vi "getPointFromLineIntersection.vi"(6 "b2":dbl, 7 "b1":dbl, 8 "error in (no error)":errorcluster, 9 "a2":dbl, 10 "a1":dbl, 11 "Utilities in":refnum<class "Utilities.lvclass">) -> (0 "error out":errorcluster, 1 "y_intersection":dbl, 2 "x_intersection":dbl, 3 "Utilities out":refnum<class "Utilities.lvclass">)   [LabVIEW 2023, in "Utilities.lvclass"]
uses:
  Utilities.lvclass
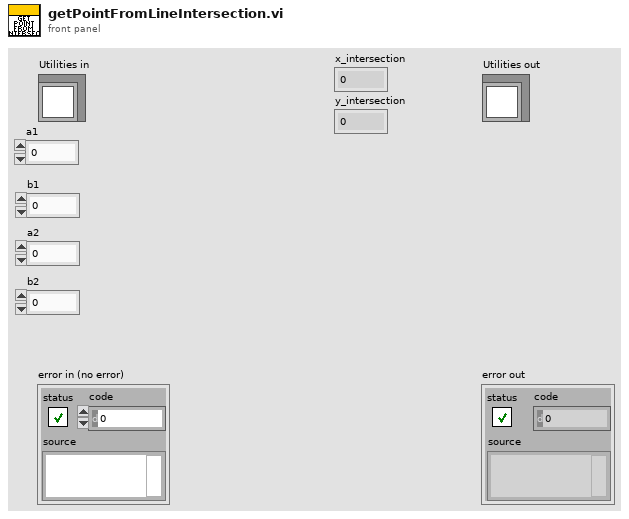
[diagram p1: front panel]
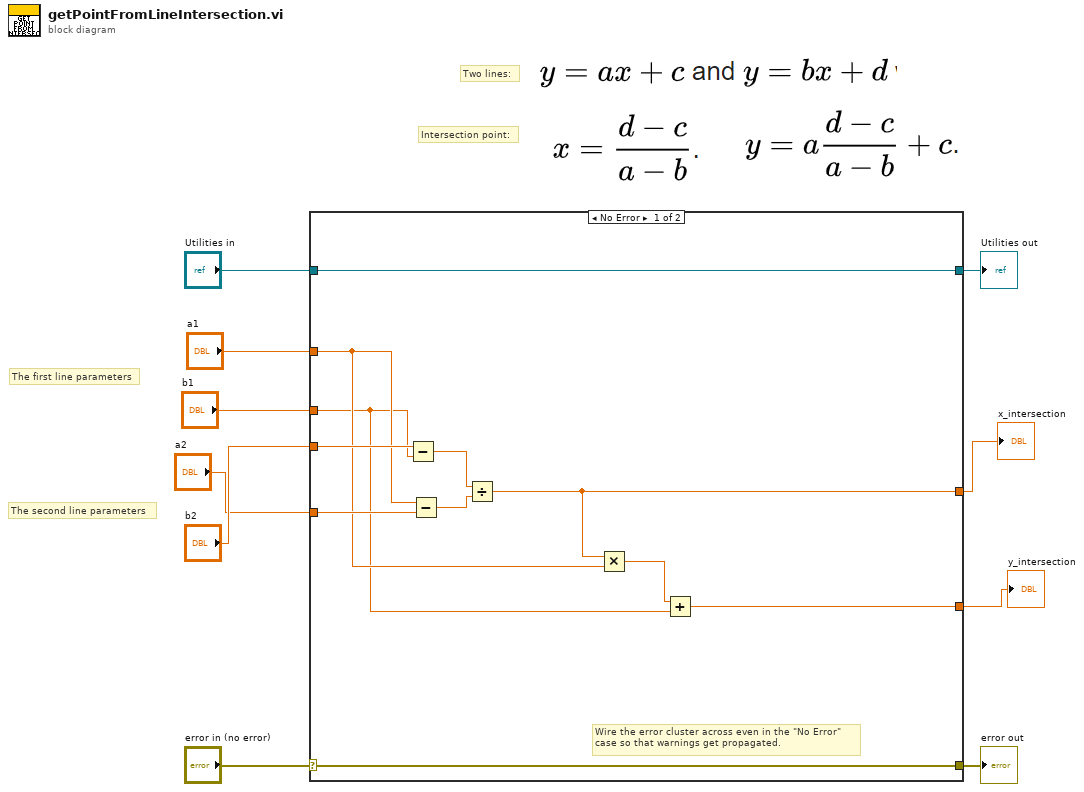
[diagram p0: block diagram]
diagram:
  # "The second line parameters"
  # "The first line parameters"
  # "Intersection point:"
  # "Two lines:"
  n1 = case shown="No Error" "error in (no error)" {
    selector: "error in (no error)" -> [w20 w23]
    tunnel: [w20 w23] -> w9
    tunnel: [w21 w22] -> w7
    tunnel: "Utilities in" -> [w21 w22]
    tunnel: "b2" -> [w19 _]
    tunnel: "b1" -> [w12 _]
    tunnel: "a1" -> [w14 _]
    tunnel: "a2" -> [w18 _]
    tunnel: [w15 _] -> w2
    tunnel: [w11 _] -> w1
    frame No Error {
      # "Wire the error cluster across even in the \"No Error\"\ncase so that warnings get propagated."
      n2 = Subtract(x=w19, y=w12) -> (x-y=w17:dbl)
      n3 = Subtract(x=w14, y=w18) -> (x-y=w16:dbl)
      n4 = Divide(x=w17, y=w16) -> (x/y=w15:dbl)
      n5 = Multiply(x=w15, y=w14) -> (x*y=w13:dbl)
      n6 = Add(x=w13, y=w12) -> (x+y=w11:dbl)
    }
    frame Error {
    }
  }
  "error out" <- w9
  "Utilities out" <- w7
  "x_intersection" <- w2
  "y_intersection" <- w1
